vi "ecg_02.vi"() -> ()   [LabVIEW 2018]
panel:
  in  "Stop Button":bool
  out "ECG":dynamicdata(graph)
  in  "Boolean":bool
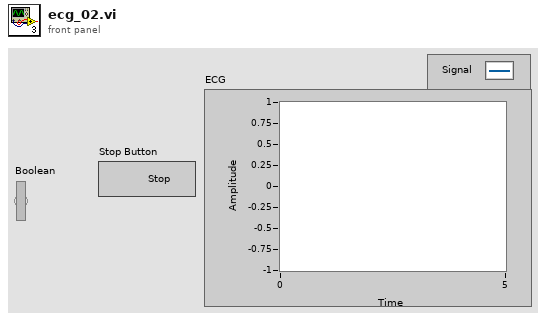
[diagram p1: front panel]
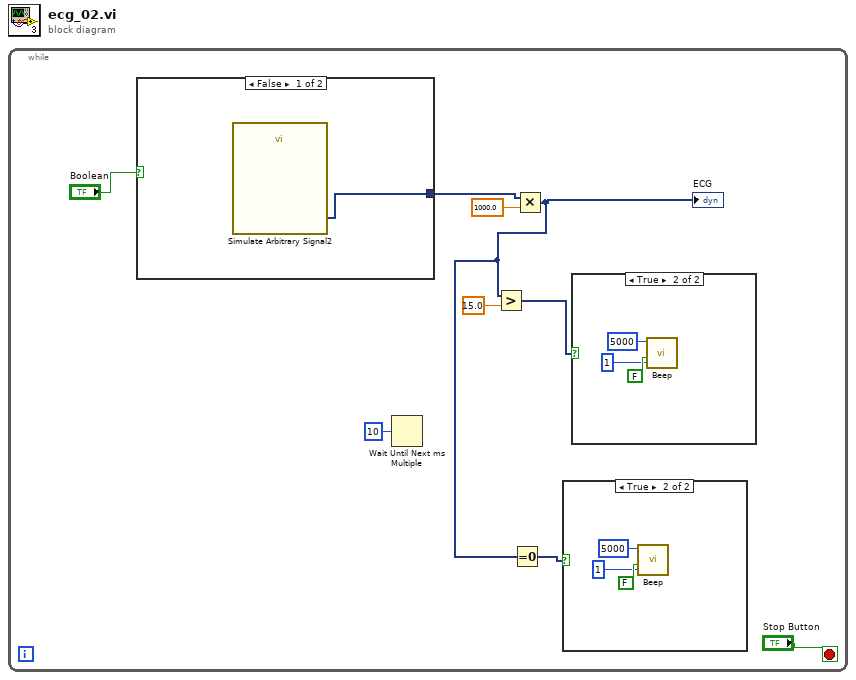
[diagram p0: block diagram]
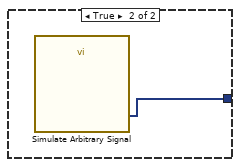
[diagram p4: hidden frame]
diagram:
  n1 = while {
    stop <- "Stop Button" stop-if-true
    n2 = case shown="False" "Boolean" {
      tunnel: [w16 w17] -> w7
      frame False {
        n3 = call "Simulate Arbitrary Signal2"() -> ("Signal"=w16:dynamicdata)  [unwired: 9 in, 2 out]
      }
      frame True {
        n4 = call "Simulate Arbitrary Signal"() -> ("Signal"=w17:dynamicdata)  [unwired: 9 in, 2 out]
      }
    }
    n5 = Wait Until Next ms Multiple(millisecond multiple=u32 10) -> ()  [unwired: 1 out]
    n6 = Multiply(x=w7, y=1000.0) -> (x*y=w2:dynamicdata)
    "ECG" <- w2
    n7 = Greater?(x=w2, y=15.0) -> (0:w5:dynamicdata)
    n8 = Equal To 0?(x=w2) -> (x = 0?=w4:dynamicdata)
    n9 = case shown="True" w4 {
      frame False {
      }
      frame True {
        n10 = call <vilib>:"Beep.vi"("use system alert? (T)"=FALSE, "duration (msec)"=u32 1, "frequency (Hz)"=u32 5000) -> ()  [unwired: 9 in]
      }
    }
    n11 = case shown="True" w5 {
      frame False {
      }
      frame True {
        n12 = call <vilib>:"Beep.vi"("use system alert? (T)"=FALSE, "duration (msec)"=u32 1, "frequency (Hz)"=u32 5000) -> ()  [unwired: 9 in]
      }
    }
  }
